vi "Enemy_Init.vi"(0 "object in":refnum<class "Enemy.lvclass">, 5 "error in (no error)":errorcluster) -> (14 "object out":refnum<class "Enemy.lvclass">, 19 "error out":errorcluster)   [LabVIEW 2021, in "Enemy.lvclass"]
uses:
  Enemy.lvclass
  D:/RoboIme/horie/SSL_AI/Team_class/Team.lvclass
  Enemy.lvclass/Enemy.ctl
  Team_class/Team.lvclass
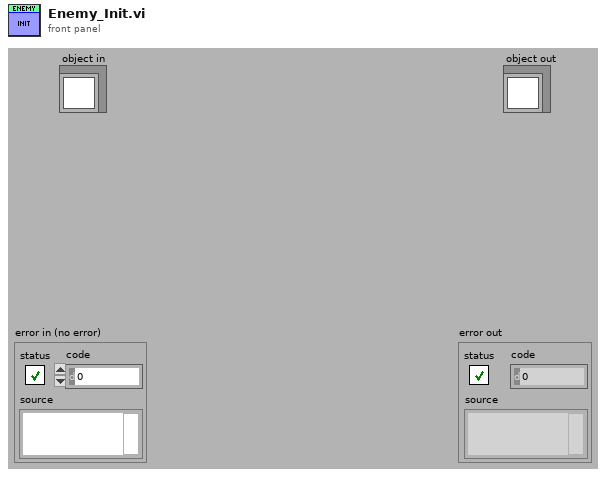
[diagram p1: front panel]
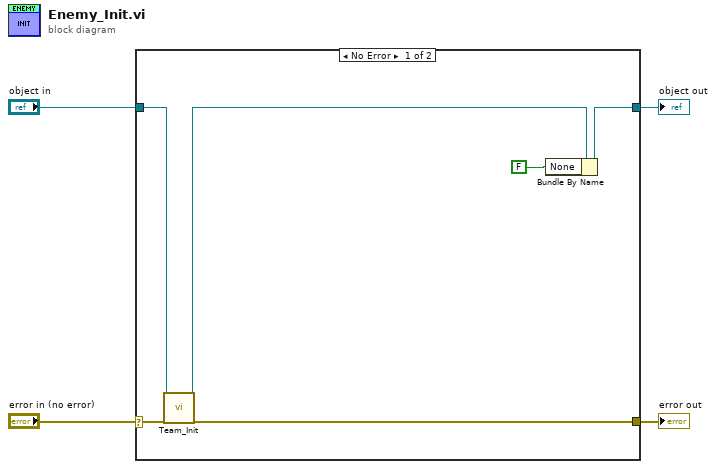
[diagram p0: block diagram]
diagram:
  n1 = case shown="No Error" "error in (no error)" {
    selector: "error in (no error)" -> [w8 w11]
    tunnel: [w10 w12] -> w4
    tunnel: "object in" -> [w6 w12]
    tunnel: [w7 w11] -> w1
    frame No Error {
      n2 = call "Team_Init.vi"("object in"=w6, "error in (no error)"=w8) -> ("object out"=w5:refnum<class "Enemy.lvclass">, "error out"=w7:errorcluster)  [unwired: 16 in]
      n3 = Bundle By Name(cluster=w5, "None"=FALSE) -> (w10:refnum<class "Enemy.lvclass">)
    }
    frame Error {
    }
  }
  "object out" <- w4
  "error out" <- w1
